vi "Save Project Documentation.vi"(8 "error in":errorcluster, 10 "Project Description":string) -> (0 "error out":errorcluster)   [LabVIEW 2019, in "Panther Dashboard.lvlib"]
doc: "_____\nCreated using DQMH Event Scripter 6.1.0.128."
uses:
  Panther Dashboard.lvlib
  Save Project Documentation Argument--cluster.ctl
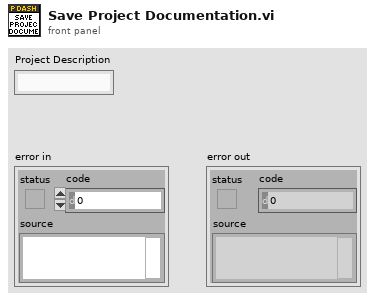
[diagram p1: front panel]
types:
  T1 = typedef "Panther Dashboard.lvlib/Save Project Documentation Argument--cluster.ctl" = cluster{"Project Description":string}
  T2 = typedef "Panther Dashboard.lvlib/Request Events--cluster.ctl" = cluster{"Stop Module":refnum<user-event>, "Show Panel":refnum<user-event>, "Hide Panel":refnum<user-event>, "Get Module Execution Status":refnum<user-event>, "Show Diagram":refnum<user-event>, "Scan DQMH Modules":refnum<user-event>, "Tree DQMH Selection":refnum<user-event>, "Open Module API Tester":refnum<user-event>, "Execute Default Event Request":refnum<user-event>, "Expand Results":refnum<user-event>, "Launch DQMH Scripting Tools":refnum<user-event>, "Generate Project Documentation":refnum<user-event>, "Set App Theme":refnum<user-event>, "Show About":refnum<user-event>, "Update Module ID":refnum<user-event>, "Save Library Description":refnum<user-event>, "Save VI Description":refnum<user-event>, "Open Documentation":refnum<user-event>, "Save Project Documentation":refnum<user-event>, "Register controls Mouse Enter":refnum<user-event>}
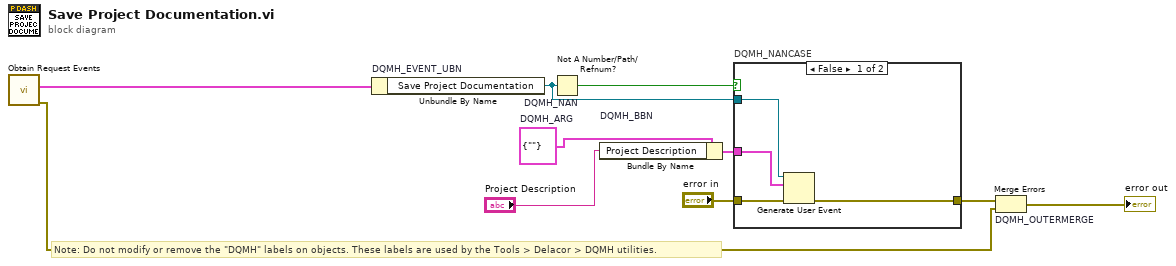
[diagram p0: block diagram]
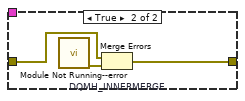
[diagram p2: hidden frame]
diagram:
  w4 = T1 {"Project Description"=""}  # DQMH_ARG
  # "Note: Do not modify or remove the \"DQMH\" labels on objects. These labels are used by the Tools > Delacor > DQMH utilities."
  n1 = call "Obtain Request Events.vi"() -> ("error out"=w2:errorcluster, "Panther Dashboard Request Events"=w1:T2)  [unwired: 10 in]
  n2 = Unbundle By Name "DQMH_EVENT_UBN"(w1) -> ("Save Project Documentation"=w6:refnum<user-event>)
  n3 = Not A Number/Path/Refnum? "DQMH_NAN"(number/path/refnum=w6) -> (NaN/Path/Refnum?=w7:bool)
  n4 = Bundle By Name "DQMH_BBN"(cluster=w4, "Project Description"="Project Description") -> (w8:T1)
  n5 = case "DQMH_NANCASE" shown="False" w7 {
    tunnel: "error in" -> [w14 w17]
    tunnel: [w13 w16] -> w5
    tunnel: w6 -> [w12 _]
    tunnel: w8 -> [w11 _]
    frame False {
      n6 = Generate User Event(user event=w12, event data cluster=w11, error in=w14) -> (error out=w13:errorcluster)  [unwired: 1 in, 1 out]
    }
    frame True {
      n7 = call "Module Not Running--error.vi"() -> ("error out"=w15:errorcluster)  [unwired: 11 in]
      n8 = Merge Errors "DQMH_INNERMERGE"(w17, w15) -> (w16:errorcluster)
    }
  }
  n9 = Merge Errors "DQMH_OUTERMERGE"(w5, w2) -> (→"error out":errorcluster)
